vi "user output.vi"(8 "error in":errorcluster, 11 "Outputs to system":T1) -> (0 "error out":errorcluster)   [LabVIEW 2014]
uses:
  output user data.ctl
  DAQmx Watchdog runtime.lvclass
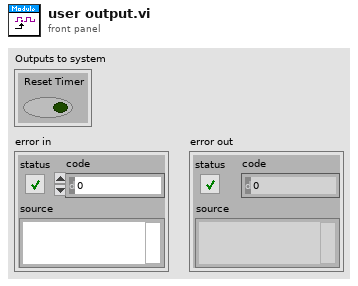
[diagram p1: front panel]
types:
  T1 = typedef "DAQmx Watchdog runtime.lvclass/output user data.ctl" = cluster{"Reset Timer":bool}
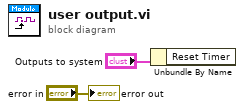
[diagram p0: block diagram]
diagram:
  n1 = Unbundle By Name("Outputs to system") -> ()  [unwired: 1 out]
  "error out" <- "error in"
